vi "Get Parameter Value Catalog.vi"(8 "error in (no error)":errorcluster {"code" format="%.0x"}, 9 "ValBufferSize":i32=2048, 10 "Name":string, 11 "instrument handle":refnum<k15>) -> (0 "error out":errorcluster {"code" format="%.0x"}, 2 "Val":string, 3 "instrument handle out":refnum<k15>)   [LabVIEW 2014, in "Agilent NA.lvlib"]
doc: "Returns a comma-separated list of valid properties values for a specific parameter name. To see the list of available parameter name please use the GetParameterCatalog() function"
uses:
  Agilent NA.lvlib
  AgNA.dll
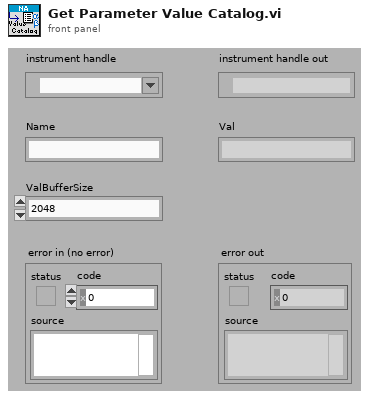
[diagram p1: front panel]
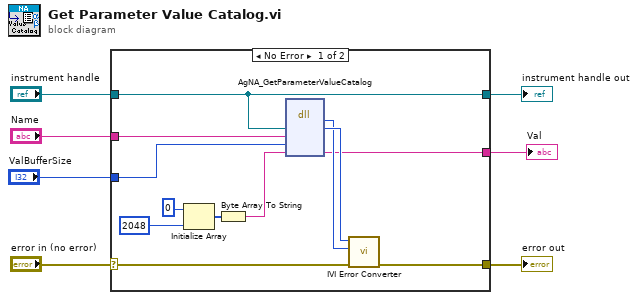
[diagram p0: block diagram]
diagram:
  n1 = case shown="No Error" "error in (no error)" {
    selector: "error in (no error)" -> [w17 w21]
    tunnel: [w16 w21] -> w7
    tunnel: "Name" -> [w15 _]
    tunnel: [w11 _] -> w4
    tunnel: "instrument handle" -> [w10 w20]
    tunnel: [w10 w20] -> w2
    tunnel: "ValBufferSize" -> [w9 _]
    frame No Error {
      n2 = Initialize Array(u8 0 ("element"), 2048 ("dimension size")) -> (w13:u8[])
      n3 = Byte Array To String(unsigned byte array=w13) -> (string=w14:string)
      n4 = dll-call lib="AgNA**.dll" fn="AgNA_GetParameterValueCatalog"("Vi"=w10, "Name"=w15, "ValBufferSize"=w9, "Val"=w14) -> (w18:i32, "Vi"=w19:u32, "Val"=w11:string)  [unwired: 5 in, 2 out]
      n5 = call "IVI Error Converter.vi"("error in (no error)"=w17, "IVI error code (0)"=w18, "instrument handle"=w19) -> ("error out"=w16:errorcluster)  [unwired: 7 in, 1 out]
    }
    frame Error {
    }
  }
  "error out" <- w7
  "instrument handle out" <- w2
  "Val" <- w4
